vi "FPGAtest.vi"() -> ()   [LabVIEW 2019]
uses:
  <vilib>/WPC Systems Ltd/GECO Driver/Lib/GECOMotion/GECOMotion/_typedefine/Axis Select.ctl
  <vilib>/WPC Systems Ltd/GECO Driver/Lib/GECOBase/GECO_Driver Class/Motion/_typedefine/GECO_Stepper Output Configuration.ctl
  <vilib>/WPC Systems Ltd/GECO Driver/Lib/GECOBase/GECO_Driver Class/Motion/_typedefine/GECO_Motion Operation Mode.ctl
  <vilib>/WPC Systems Ltd/GECO Driver/Lib/GECOBase/GECO_Driver Class/GECO_SlotName.ctl
  <vilib>/WPC Systems Ltd/GECO Driver/Lib/GECOBase/GECO_Driver Class/Motion/_typedefine/GECO_ActiveHighLow.ctl
  <vilib>/WPC Systems Ltd/GECO Driver/GECODriver/GECO_Initialize_RT/Initialize VIs/Initialize_GECOUnoRT_4HX.vi
  <vilib>/WPC Systems Ltd/GECO Driver/Lib/GECOBase/GECO_Driver Class/GECO_Driver.lvclass
  <vilib>/WPC Systems Ltd/GECO Driver/Lib/GECOMotion/GECOMotion/GECO Motion.lvclass
panel:
  in  "Reverse Polarity":T1=enum."Active Low"
  in  "Forward Polarity":T1=enum."Active Low"
  in  "Motion Controller Slot":T2
  in  "Motion Operation Mode":T3
  in  "Deacceleration (100000)":u32=100000
  in  "Acceleration (100000)":u32=100000
  in  "Velocity (10000)":i32=10000 min=-20000000 max=20000000
  in  "Target Position (0)":i32=1000
  in  "Reverse Enable?":bool
  in  "Forward Enable?":bool=TRUE
  in  "Stepper Output Configuration":T4
  in  "Axis Select":T5
  in  "Stop Move":bool
  out "Move Complete?":bool
  out "Logical Position":i32
  out "Encoder Position":i32
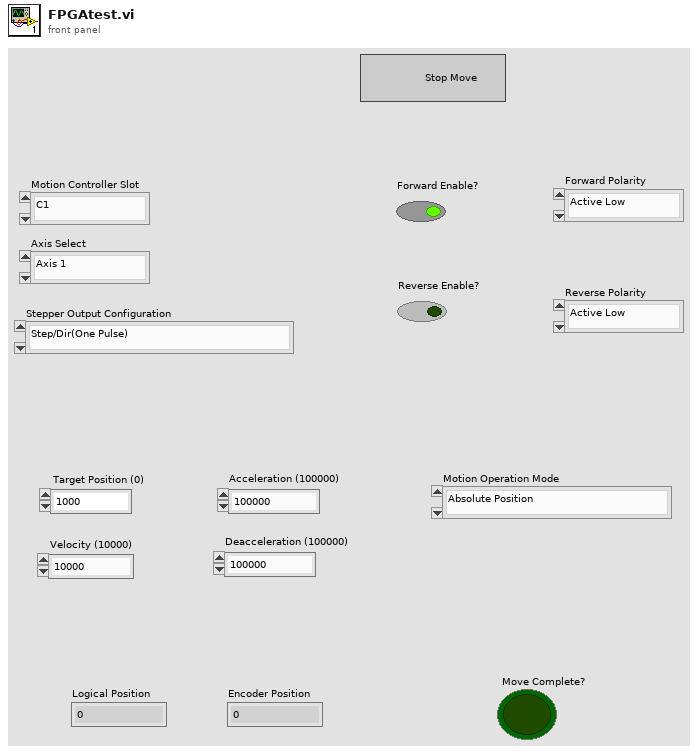
[diagram p1: front panel]
types:
  T1 = typedef "GECO_Driver.lvclass/GECO_ActiveHighLow.ctl" = enum16{"Active High", "Active Low"}
  T2 = typedef "GECO_Driver.lvclass/GECO_SlotName.ctl" = enum16{"C1", "C2", "C3", "C4"}
  T3 = typedef "GECO_Driver.lvclass/GECO_Motion Operation Mode.ctl" = enum16{"Absolute Position", "Relative Position", "Velocity"}
  T4 = typedef "GECO_Driver.lvclass/GECO_Stepper Output Configuration.ctl" = enum16{"Step/Dir(One Pulse)", "CW/CCW(Two Pulse)"}
  T5 = typedef "GECO Motion.lvclass/Axis Select.ctl" = enum16{"Axis 1", "Axis 2", "Axis 3", "Axis 4"}
  T6 = cluster{"Forward Enable":bool, "Forward Polarity":T1}
  T7 = cluster{"Reverse Enable":bool, "Reverse Polarity":T1}
  T8 = cluster{"Motion Operation Mode":T3, "Target Position (0)":i32, "Velocity (10000)":i32, "Acceleration (100000)":u32, "Deacceleration (100000)":u32}
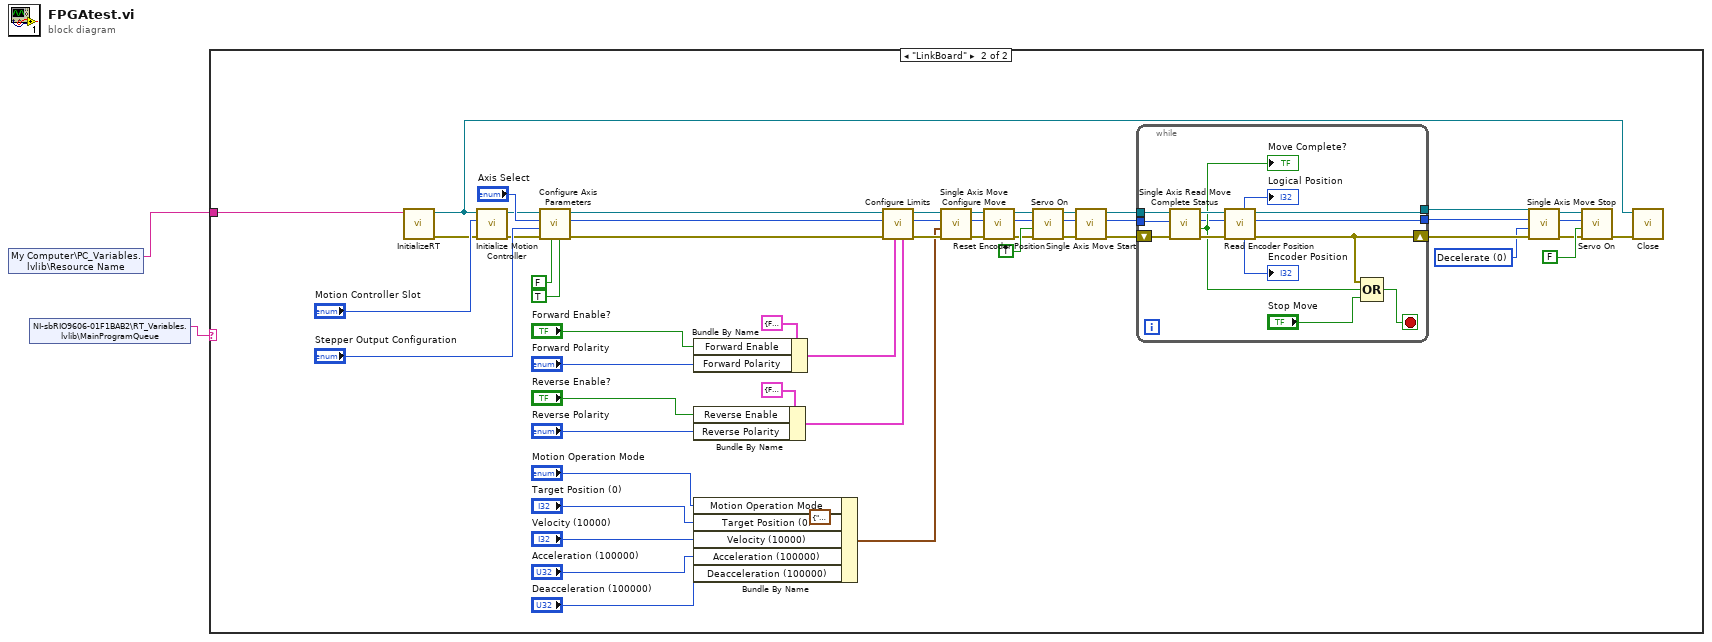
[diagram p0: block diagram]
diagram:
  n1 = shared-variable "My Computer\\PC_Variables.lvlib\\Resource Name"() -> (w1:tag)  [unwired: 1 in, 1 out]
  n2 = shared-variable "NI-sbRIO9606-01F1BAB2\\RT_Variables.lvlib\\MainProgramQueue"() -> (w2:string)  [unwired: 1 in, 1 out]
  n3 = case shown="\"LinkBoard\"" w2 {
    tunnel: w1 -> [_ w3]
    frame "False", Default {
    }
    frame "LinkBoard" {
      w48 = u16 0 items=["Decelerate", "Halt"] ("Motion Stop Type")
      n4 = call-poly <vilib>:"InitializeRT.vi"("resource name"=w3) -> ("error out"=w22:errorcluster, "GECO_Driver out"=w20:refnum<class "GECO_Driver.lvclass">)  [unwired: 9 in]
      n5 = call <vilib>:"Initialize Motion Controller.vi"("error in (no error)"=w22, "Slot"="Motion Controller Slot", "GECO_Driver in"=w20) -> ("error out"=w21:errorcluster, "Motion reference out"=w23:refnum<class "GECO Motion.lvclass">)  [unwired: 7 in]
      n6 = call <vilib>:"Configure Axis Parameters.vi"("Reverse Encoder Direction?"=TRUE ("Encoder Direction"), "Reverse Axis Direction?"=FALSE ("Axis Direction"), "error in (no error)"=w21, "Stepper Output Configuration"="Stepper Output Configuration", "Axis Select"="Axis Select", "GECO Motion in"=w23) -> ("error out"=w40:errorcluster, "Axis Select out"=w11:T5, "GECO Motion out"=w41:refnum<class "GECO Motion.lvclass">)  [unwired: 3 in]
      n7 = Bundle By Name(cluster=T6 {"Forward Enable"=FALSE, "Forward Polarity"=enum."Active Low"} ("Forward"), "Forward Enable"="Forward Enable?", "Forward Polarity"="Forward Polarity") -> (w18:T6)
      n8 = Bundle By Name(cluster=T7 {"Reverse Enable"=FALSE, "Reverse Polarity"=enum."Active Low"} ("Reverse"), "Reverse Enable"="Reverse Enable?", "Reverse Polarity"="Reverse Polarity") -> (w14:T7)
      n9 = Bundle By Name(cluster=T8 {"Motion Operation Mode"=enum."Absolute Position", "Target Position (0)"=0, "Velocity (10000)"=10000, "Acceleration (100000)"=100000, "Deacceleration (100000)"=100000} ("Singel Axis Move Paramters"), "Motion Operation Mode"="Motion Operation Mode", "Target Position (0)"="Target Position (0)", "Velocity (10000)"="Velocity (10000)", "Acceleration (100000)"="Acceleration (100000)", "Deacceleration (100000)"="Deacceleration (100000)") -> (w34:T8)
      n10 = call <vilib>:"Configure Limits.vi"("Reverse"=w14, "Forward"=w18, "error in (no error)"=w40, "Axis Select"=w11, "GECO Motion in"=w41) -> ("error out"=w38:errorcluster, "Axis Select out"=w10:T5, "GECO Motion out"=w39:refnum<class "GECO Motion.lvclass">)  [unwired: 4 in]
      n11 = call <vilib>:"Single Axis Move Configure Move.vi"("error in (no error)"=w38, "Singel Axis Move Paramters"=w34, "Axis Select"=w10, "GECO Motion in"=w39) -> ("error out"=w36:errorcluster, "Axis Select out"=w9:T5, "GECO Motion out"=w37:refnum<class "GECO Motion.lvclass">)  [unwired: 5 in]
      n12 = call <vilib>:"Reset Encoder Position.vi"("error in (no error)"=w36, "Axis Select"=w9, "GECO Motion in"=w37) -> ("error out"=w42:errorcluster, "Axis Select out"=w8:T5, "GECO Motion out"=w43:refnum<class "GECO Motion.lvclass">)  [unwired: 6 in]
      n13 = call <vilib>:"Servo On.vi"("error in (no error)"=w42, "Servo On"=TRUE, "Axis Select"=w8, "GECO Motion in"=w43) -> ("error out"=w53:errorcluster, "Axis Select out"=w7:T5, "GECO Motion out"=w54:refnum<class "GECO Motion.lvclass">)  [unwired: 5 in]
      n14 = call <vilib>:"Single Axis Move Start.vi"("error in (no error)"=w53, "Axis Select"=w7, "GECO Motion in"=w54) -> ("error out"=w51:errorcluster, "Axis Select out"=w6:T5, "GECO Motion out"=w52:refnum<class "GECO Motion.lvclass">)  [unwired: 6 in]
      n15 = while {
        tunnel: w52 -> [w62]
        tunnel: [w67] -> w50
        shift-right: [w64] -> w49
        shift-left: w51 -> [w63]
        tunnel: w6 -> [w58]
        tunnel: [w56] -> w5
        stop <- w68 stop-if-true
        n16 = call <vilib>:"Single Axis Read Move Complete Status.vi"("error in (no error)"=w63, "Axis Select"=w58, "GECO Motion in"=w62) -> ("error out"=w65:errorcluster, "Move Complete?"=w61:bool, "Axis Select out"=w57:T5, "GECO Motion out"=w66:refnum<class "GECO Motion.lvclass">)  [unwired: 5 in]
        "Move Complete?" <- w61
        n17 = call <vilib>:"Read Encoder Position.vi"("error in (no error)"=w65, "Axis Select"=w57, "GECO Motion in"=w66) -> ("error out"=w64:errorcluster, "Axis Select out"=w56:T5, "GECO Motion out"=w67:refnum<class "GECO Motion.lvclass">, "Encoder Position"=→"Encoder Position":i32, "Logical Position"=→"Logical Position":i32)  [unwired: 4 in]
        n18 = Compound Arithmetic op=OR(w64, w61, "Stop Move") -> (w68:bool)
      }
      n19 = call <vilib>:"Single Axis Move Stop.vi"("error in (no error)"=w49, "Motion Stop Type"=w48, "Axis Select"=w5, "GECO Motion in"=w50) -> ("error out"=w45:errorcluster, "Axis Select out"=w4:T5, "GECO Motion out"=w46:refnum<class "GECO Motion.lvclass">)  [unwired: 5 in]
      n20 = call <vilib>:"Servo On.vi"("error in (no error)"=w45, "Servo On"=FALSE, "Axis Select"=w4, "GECO Motion in"=w46) -> ("error out"=w44:errorcluster)  [unwired: 5 in, 2 out]
      n21 = call <vilib>:"Close.vi"("error in (no error)"=w44, "GECO_Driver in"=w20) -> ()  [unwired: 9 in, 1 out]
    }
  }
